vi "user32_TileWindows.vi"(0 "hWndParent":u32, 1 "wHow":u32(ring) items=["VERTICAL"=0, "HORIZONTAL"=1, "SKIPDISABLED"=2, "ZORDER"=4], 5 "lpRect":T1, 7 "cKids":u32, 9 "lpKids":u32, 11 "错误输入（无错误）":errorcluster) -> (4 "dup hWndParent":u32, 6 "ArrangedWindowNum":i32, 15 "错误输出":errorcluster)   [LabVIEW 2011]
doc: "Tiles the specified child windows of the specified parent window.\n\nhttp://msdn.microsoft.com/en-us/library/windows/desktop/ms633554(v=vs.85).aspx"
uses:
  user32.dll
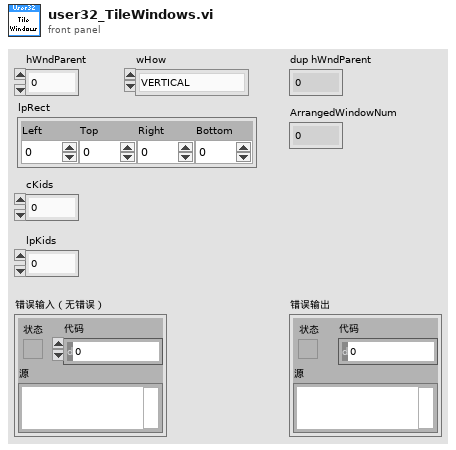
[diagram p1: front panel]
types:
  T1 = cluster{"Left":i32, "Top":i32, "Right":i32, "Bottom":i32}
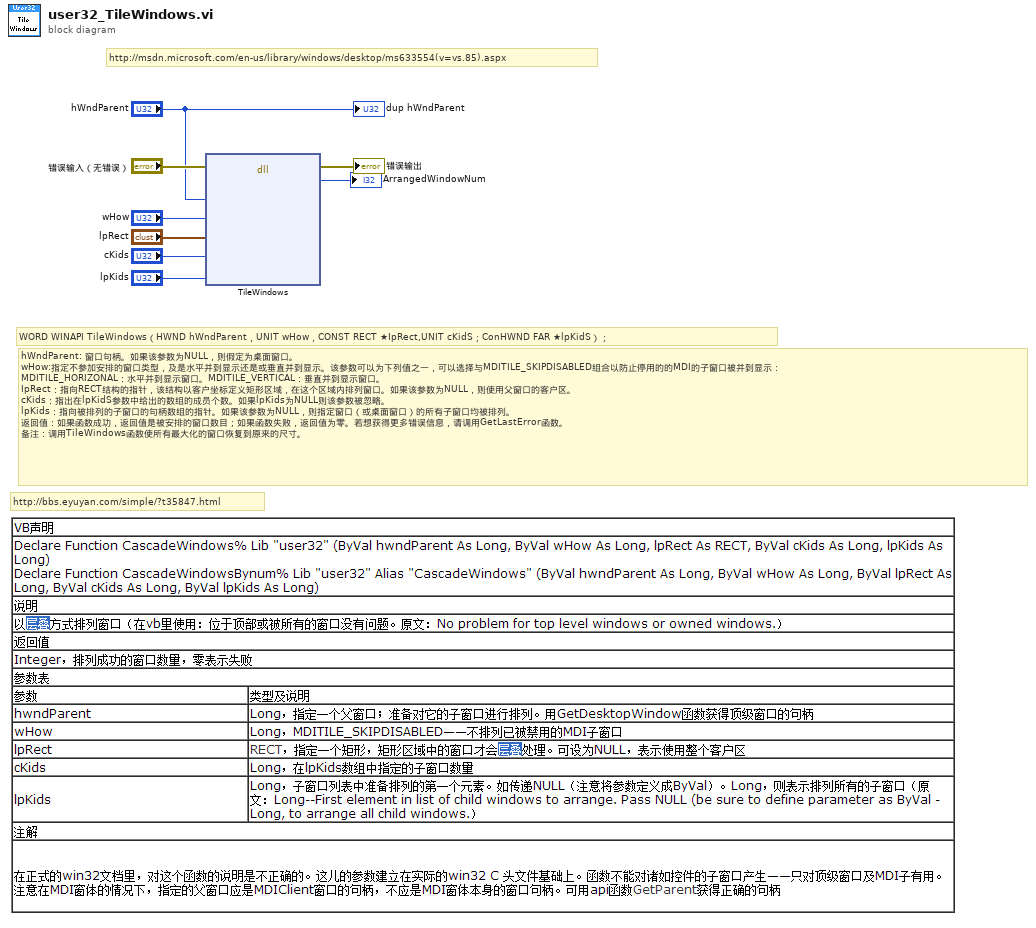
[diagram p0: block diagram]
diagram:
  # "http://msdn.microsoft.com/en-us/library/windows/desktop/ms633554(v=vs.85).aspx"
  # "http://bbs.eyuyan.com/simple/?t35847.html"
  # "hWndParent: 窗口句柄。如果该参数为NULL，则假定为桌面窗口。\nwHow:指定不参加安排的窗口类型，及是水平并到显示还是或垂直并到显示。该参数可以为下列值之一，可以选择与MDITILE_SKIPDISABLED组合以防止停用的的MDI的子窗口被并到显示：\nMDITILE_HORIZONAL：水平并到显示窗口。MDITILE_VERTICAL：垂直并到显示窗口。\nIpRect：指向RECT结构的指针，该结构以客户坐标定义矩形区域，在这个区域内排列窗口。如果该参数为NULL，则使用父窗口的客户区。\ncKids：指出在lpKidS参数中给出的数组的成员个数。如果lpKids为NULL则该参数被忽略。\nlpKids：指向被排列的子窗口的句柄数组的指针。如果该参数为NULL，则指定窗口（或桌面窗口）的所有子窗口均被排列。\n返回值：如果函数成功，返回值是被安排的窗口数目；如果函数失败，返回值为零。若想获得更多错误信息，请调用GetLastError函数。\n备注：调用TileWindows函数使所有最大化的窗口恢复到原来的尺寸。"
  # "WORD WINAPI TileWindows（HWND hWndParent，UNIT wHow，CONST RECT ★IpRect,UNIT cKidS；ConHWND FAR ★lpKidS）；"
  n1 = dll-call lib="user32.dll" fn="TileWindows"(error in="错误输入（无错误）", "hWndParent"="hWndParent", "wHow"="wHow", "lpRect"="lpRect", "cKids"="cKids", "lpKids"="lpKids") -> (error out=→"错误输出":errorcluster, "ArrangedWNum"=→"ArrangedWindowNum":i32)  [unwired: 7 in, 1 out]
  "dup hWndParent" <- "hWndParent"
